vi "TimeShiftFocii.vi"(0 "Array data":dbl[][](array[numeric]), 1 "ZoneStart":sgl[](array[numeric]), 2 "ZoneShift":sgl[](array[numeric]), 3 "ZoneLength":sgl[](array[numeric]), 4 "IndexVals":sgl[](array[numeric]), 6 "attn_dB":sgl, 8 "Scale Voltage?":bool=TRUE, 9 "A/D info.# A/D bits":u16) -> (19 "Synth App Out":dbl[][](array[numeric]))   [LabVIEW 2022 SP3]
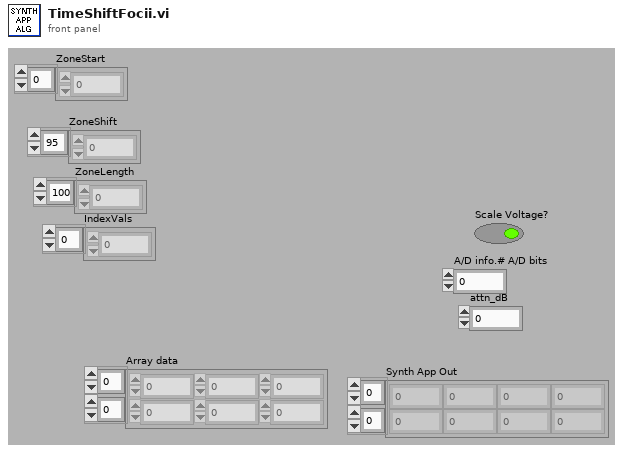
[diagram p1: front panel]
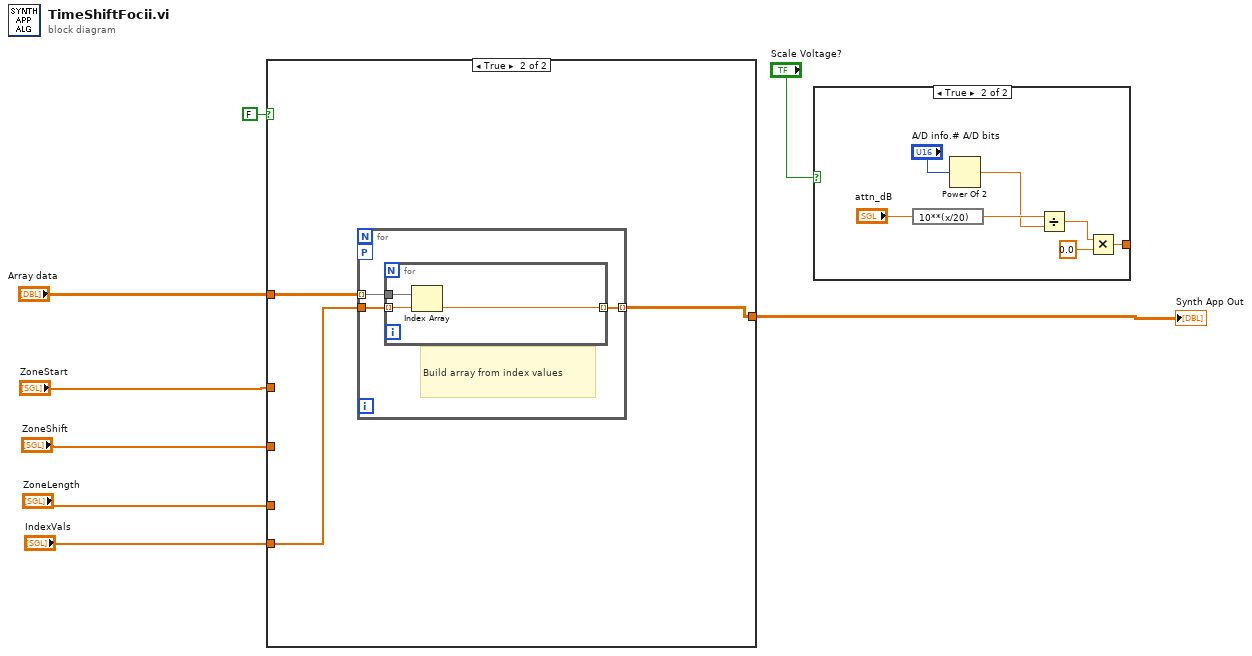
[diagram p0: block diagram]
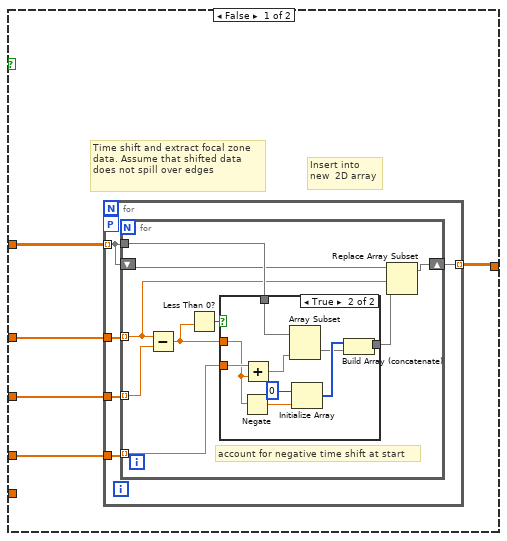
[diagram p2: hidden frame]
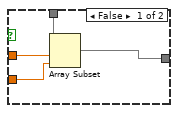
[diagram p3: hidden frame]
diagram:
  n1 = case shown="True" FALSE {
    tunnel: "ZoneShift" -> [w11 _]
    tunnel: "ZoneLength" -> [w10 _]
    tunnel: "ZoneStart" -> [w12 _]
    tunnel: [w9 w43] -> w3
    tunnel: "Array data" -> [w13 w42]
    tunnel: "IndexVals" -> [_ w41]
    frame False {
      # "Time shift and extract focal zone data. Assume that shifted data does not spill over edges"
      # "Insert into new  2D array"
      n2 = for {
        tunnel: w13 -> [w14] mode=indexing
        tunnel: w12 -> [w18]
        tunnel: w11 -> [w17]
        tunnel: w10 -> [w16]
        tunnel: [w15] -> w9 mode=indexing
        workers-P: _ -> [_]
        n3 = for {
          tunnel: w18 -> [w20] mode=indexing
          tunnel: w16 -> [w27] mode=indexing
          tunnel: w17 -> [w26] mode=indexing
          tunnel: w14 -> [w23]
          shift-right: [w22] -> w15
          shift-left: w14 -> [w21]
          # "account for negative time shift at start"
          n4 = Subtract(x=w20, y=w26) -> (x-y=w24:sgl)
          n5 = Less Than 0?(x=w24) -> (x < 0?=w25:bool)
          n6 = case shown="True" w25 {
            tunnel: w23 -> [w31 w39]
            tunnel: w27 -> [w29 w40]
            tunnel: [w30 w34] -> w19
            tunnel: w24 -> [w28 w37]
            frame False {
              n7 = Array Subset(array=w31, index=w28, length=w29) -> (w30:dbl[])
            }
            frame True {
              n8 = Negate(x=w37) -> (-x=w32:sgl)
              n9 = Add(x=w40, y=w37) -> (x+y=w33:sgl)
              n10 = Array Subset(array=w39, length=w33) -> (w35:dbl[])  [unwired: 1 in]
              n11 = Initialize Array(i16 0, w32) -> (w36:i16[])
              n12 = Build Array (concatenate)(w36, w35) -> (w34:dbl[])
            }
          }
          n13 = Replace Array Subset(array=w21, new element=w19, index=w20) -> (w22:dbl[])
        }
      }
    }
    frame True {
      n14 = for {
        tunnel: w42 -> [w46] mode=indexing
        tunnel: [w45] -> w43 mode=indexing
        workers-P: _ -> [_]
        tunnel: w41 -> [w44]
        # "Build array from index values"
        n15 = for {
          tunnel: w46 -> [w49]
          tunnel: [w48] -> w45 mode=indexing
          tunnel: w44 -> [w47] mode=indexing
          n16 = Index Array(array=w49, index=w47) -> (element=w48:dbl)
        }
      }
    }
  }
  "Synth App Out" <- w3
  n17 = case shown="True" "Scale Voltage?" {
    tunnel: [_ w56] -> _
    frame False {
    }
    frame True {
      n18 = expression code="10**(x/20)"("attn_dB") -> (w54:sgl)
      n19 = Power Of 2(x="A/D info.# A/D bits") -> (2^x=w51:dbl)
      n20 = Divide(x=w54, y=w51) -> (x/y=w53:dbl)
      n21 = Multiply(x=w53, y=0.0) -> (x*y=w56:dbl)
    }
  }
